vi "Parameter.vi"(5 "继承模式":string, 7 "模式":enum16{"select", "insert", "update", "delete"}(ring), 8 "nameData":T2(array[cluster]), 10 "parameterName":string, 11 "productsName":string) -> (0 "data":string[][](array[string]))   [LabVIEW 2013]
uses:
  <vilib>/Utility/VariantDataType/Type.ctl
  <vilib>/addons/database/_DB Variant To Data/Database Variant To Data.xnode
  <vilib>/Utility/VariantDataType/VariantType.lvlib
panel:
  out "SQL query":string
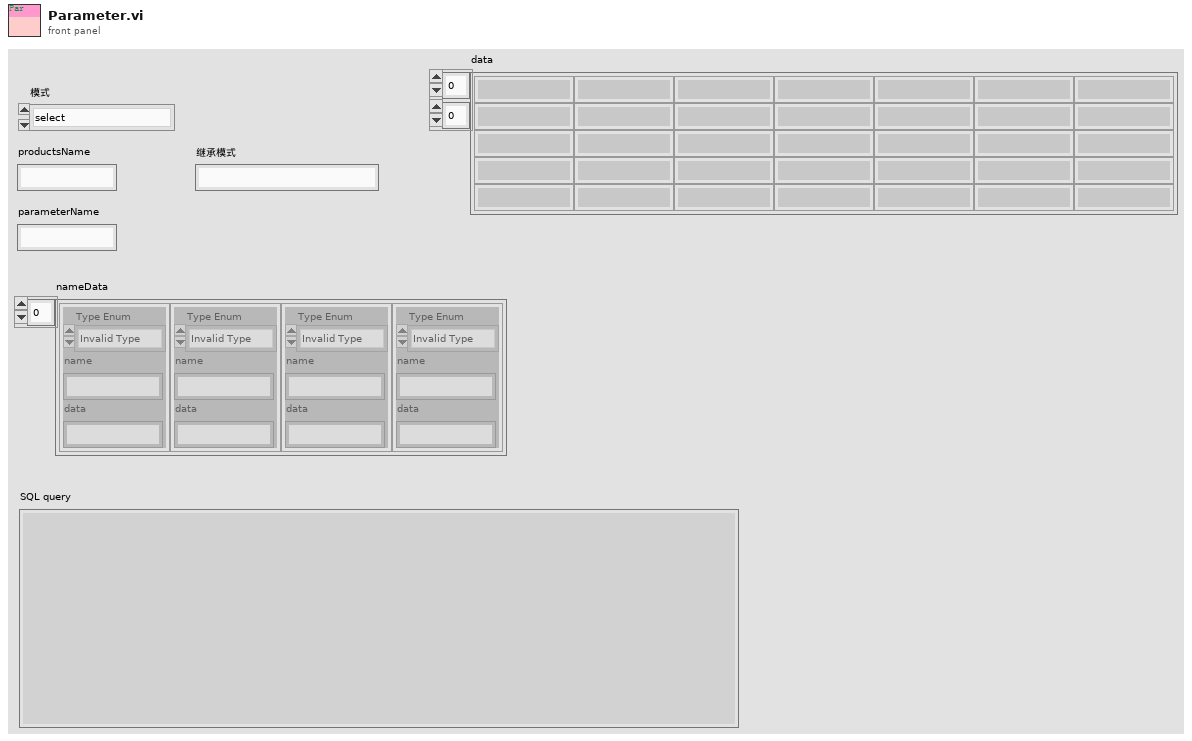
[diagram p1: front panel]
types:
  T1 = typedef "VariantType.lvlib/Type.ctl" = enum8{"Invalid Type", "Void", "I8", "I16", "I32", "I64", "U8", "U16", "U32", "U64", "Single Float", "Double Float", "Extended Float", "Single Complex", "Double Complex", "Extended Complex", "Enum U8", "Enum U16", "Enum U32", "Enum U64", "Single Float With Unit", "Double Float With Unit", "Extended Float With Unit", "Single Complex with Unit", "Double Complex with Unit", "Extended Complex with Unit", "Boolean", "String", "Path", "Picture", "Tag", "Array", "Cluster", "Variant", "LV Variant", "Waveform", "Timestamp", "Digital Waveform", "Digital Data", "ExpressData", "Refnum", "External Data", "VI", "Poly VI", "LabVIEW Class Instance", "Fixed Point"}
  T2 = cluster{"Type Enum":T1, "name":string, "data":string}[]
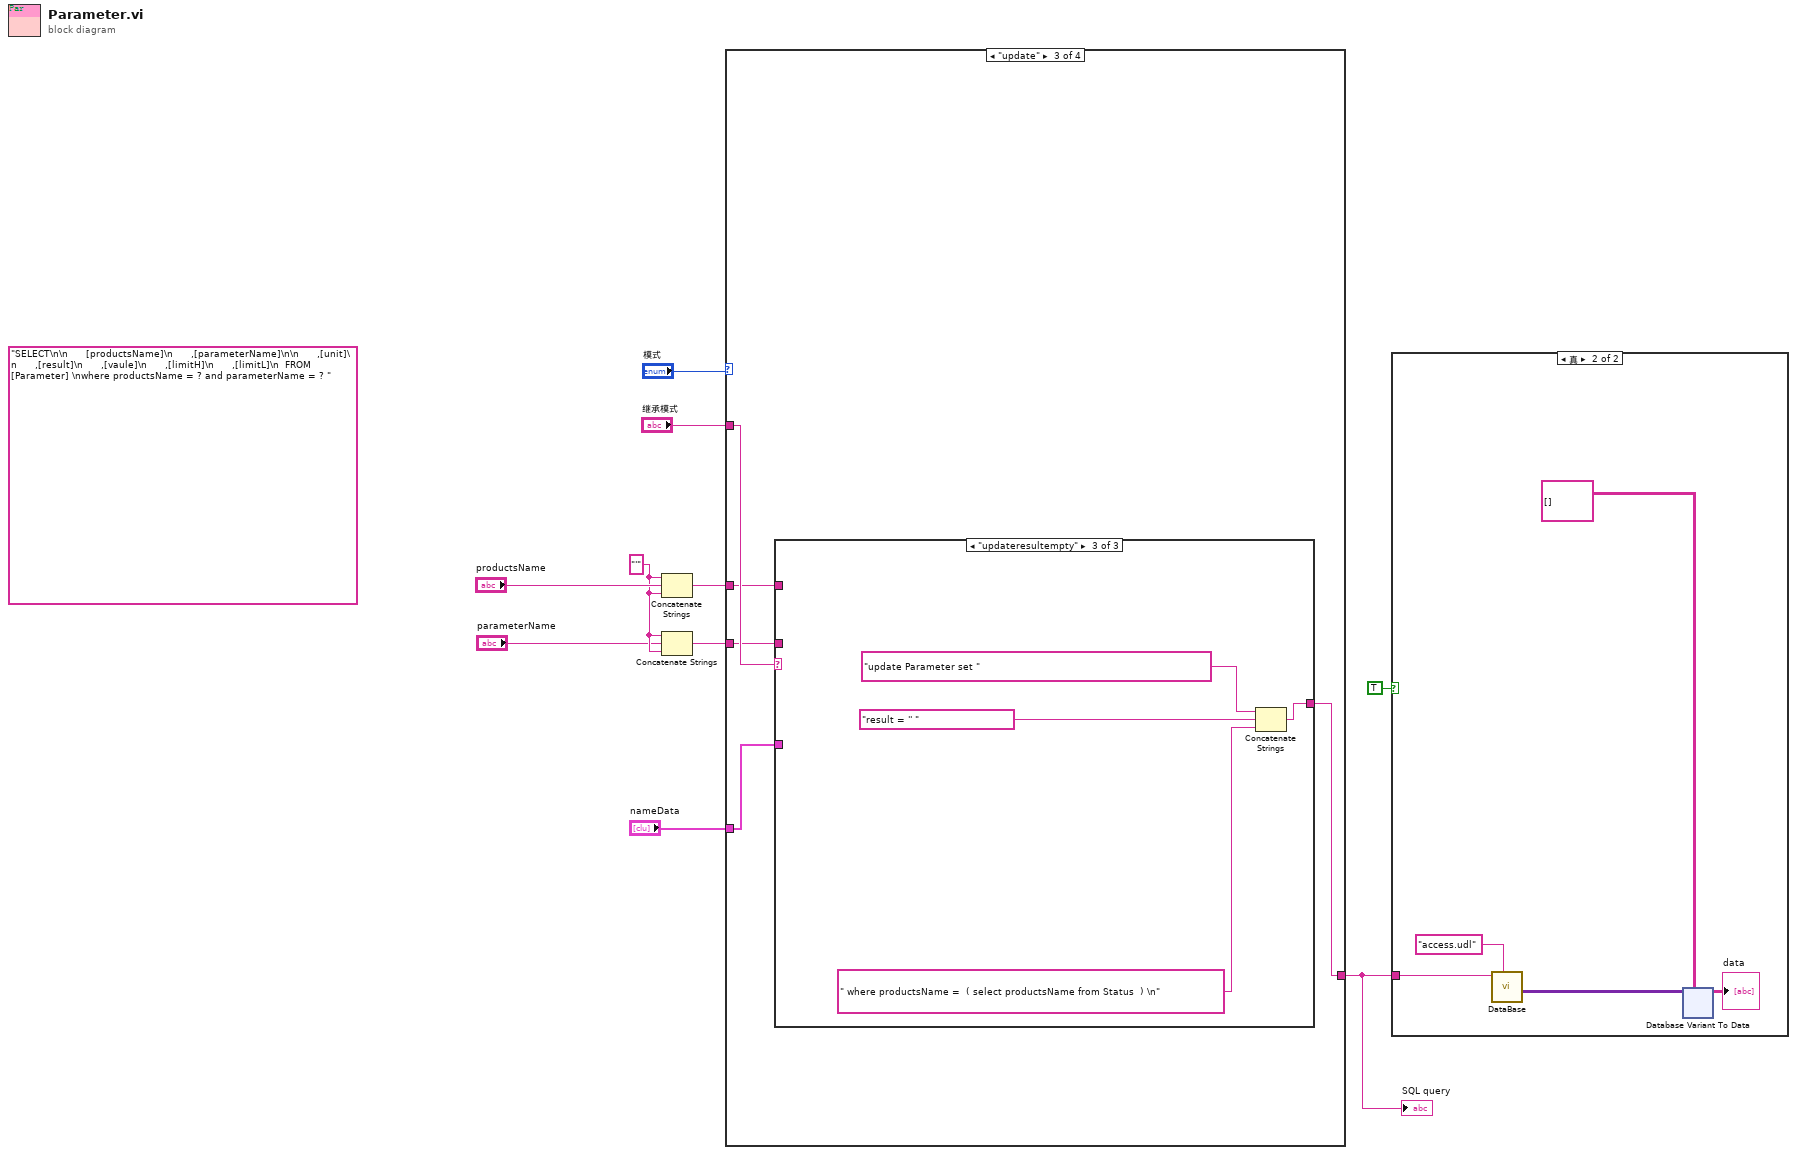
[diagram p0: block diagram]
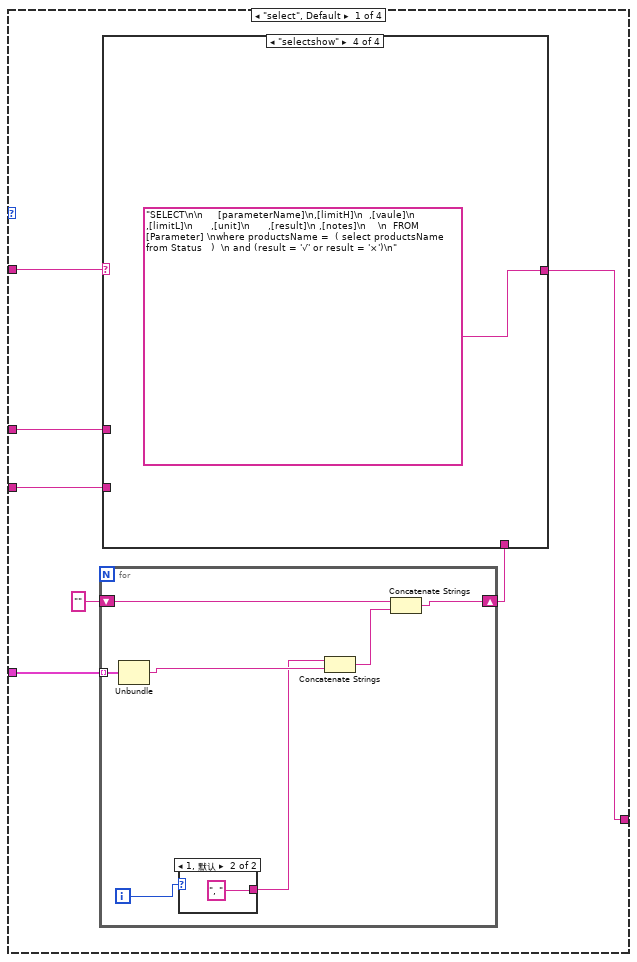
[diagram p3: hidden frame]
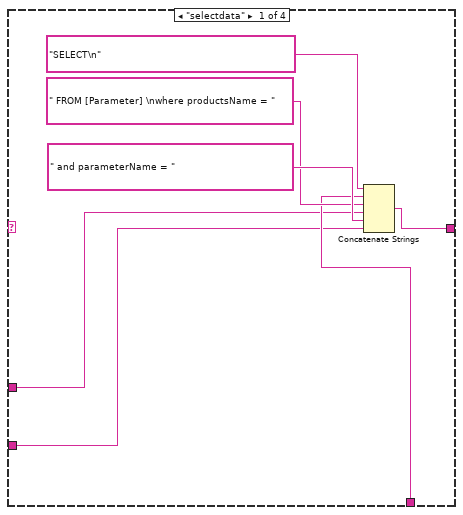
[diagram p4: hidden frame]
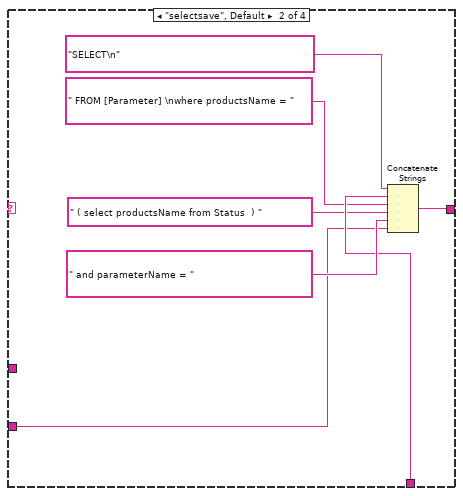
[diagram p5: hidden frame]
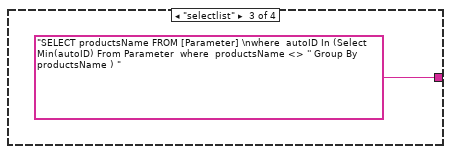
[diagram p6: hidden frame]
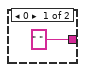
[diagram p7: hidden frame]
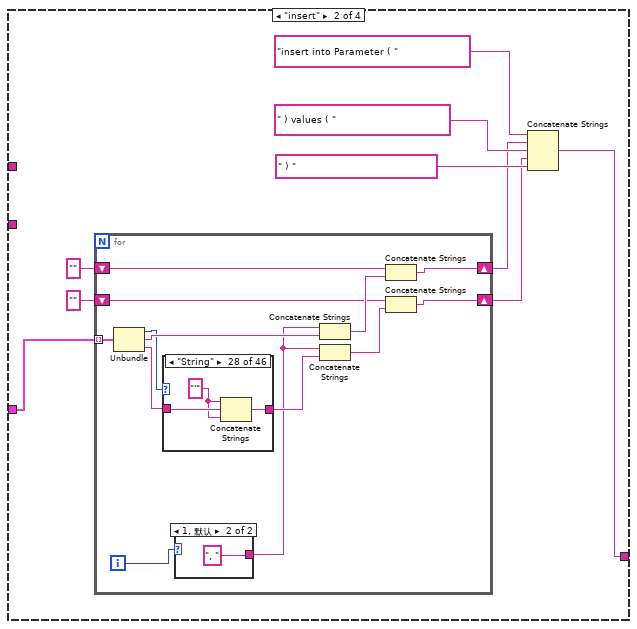
[diagram p8: hidden frame]
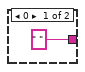
[diagram p9: hidden frame]
diagram:
  w4 = "'" ("字符串")
  (unwired) "SELECT\n\n      [productsName]\n      ,[parameterName]\n\n      ,[unit]\n      ,[result]\n      ,[vaule]\n      ,[limitH]\n      ,[limitL]\n  FROM [Parameter] \nwhere productsName = ? and parameterName = ? " ("SQL query")
  n1 = Concatenate Strings(w4, "productsName", w4) -> (w6:string)
  n2 = Concatenate Strings(w4, "parameterName", w4) -> (w2:string)
  n3 = case shown="\"update\"" "模式" {
    tunnel: [w11 w43 w77 w137] -> w9
    tunnel: "nameData" -> [w16 w49 w76 _]
    tunnel: w6 -> [w13 _ w73 w138]
    tunnel: w2 -> [w12 _ w74 _]
    tunnel: "继承模式" -> [w15 _ w75 _]
    frame "select", Default {
      n4 = for {
        tunnel: w16 -> [w40] mode=indexing
        shift-right: [w38] -> w14
        shift-left: "" ("SQL query") -> [w39]
        i -> [w35]
        n5 = Unbundle(w40) -> ("name"=w36:string)  [unwired: 2 out]
        n6 = case shown="1, 默认" w35 {
          tunnel: [" " ("字符串") ", " ("字符串")] -> w34
          frame 0 {
          }
          frame 1, Default {
          }
        }
        n7 = Concatenate Strings(w34, w36) -> (w37:string)
        n8 = Concatenate Strings(w39, w37) -> (w38:string)
      }
      n9 = case shown="\"selectshow\"" w15 {
        tunnel: [w18 w25 "SELECT productsName FROM [Parameter] \nwhere  autoID In (Select Min(autoID) From Parameter  where  productsName <> '' Group By productsName ) " ("SQL query") "SELECT\n\n     [parameterName]\n,[limitH]\n  ,[vaule]\n      ,[limitL]\n      ,[unit]\n      ,[result]\n ,[notes]\n    \n  FROM [Parameter] \nwhere productsName =  ( select productsName from Status   )  \n and (result = '√' or result = '×')\n" ("SQL query")] -> w11
        tunnel: w14 -> [w21 w29 _ _]
        tunnel: w13 -> [w20 _ _ _]
        tunnel: w12 -> [w19 w26 _ _]
        frame "selectdata" {
          n10 = Concatenate Strings("SELECT\n" ("SQL query"), w21, " FROM [Parameter] \nwhere productsName = " ("SQL query"), w20, " and parameterName = " ("SQL query"), w19) -> (w18:string)
        }
        frame "selectsave", Default {
          n11 = Concatenate Strings("SELECT\n" ("SQL query"), w29, " FROM [Parameter] \nwhere productsName = " ("SQL query"), " ( select productsName from Status  ) " ("SQL query"), " and parameterName = " ("SQL query"), w26) -> (w25:string)
        }
        frame "selectlist" {
        }
        frame "selectshow" {
        }
      }
    }
    frame "insert" {
      n12 = for {
        tunnel: w49 -> [w64] mode=indexing
        shift-right: [w62] -> w45
        shift-left: "" ("SQL query") -> [w63]
        shift-right: [w59] -> w44
        shift-left: "" ("SQL query") -> [w60]
        i -> [w53]
        n13 = Unbundle(w64) -> ("Type Enum"=w56:T1, "name"=w57:string, "data"=w55:string)
        n14 = case shown="\"String\"" w56 {
          tunnel: w55 -> [w67 _ _ _ _ _ _ _ _ _ w68 w69 _ _ _ _ _ _ _ _ _ _ _ _ _ _ _ w72 _ _ _ _ _ _ _ _ _ _ _ _ _ _ _ _ _ _]
          tunnel: [w67 _ _ _ _ _ _ _ _ _ w68 w69 _ _ _ _ _ _ _ _ _ _ _ _ _ _ _ w70 _ _ _ _ _ _ _ _ _ _ _ _ _ _ _ _ _ _] -> w54
          frame "Invalid Type", Default {
          }
          frame "Void" {
          }
          frame "I8" {
          }
          frame "I16" {
          }
          frame "I32" {
          }
          frame "I64" {
          }
          frame "U8" {
          }
          frame "U16" {
          }
          frame "U32" {
          }
          frame "U64" {
          }
          frame "Single Float" {
          }
          frame "Double Float" {
          }
          frame "Extended Float" {
          }
          frame "Single Complex" {
          }
          frame "Double Complex" {
          }
          frame "Extended Complex" {
          }
          frame "Enum U8" {
          }
          frame "Enum U16" {
          }
          frame "Enum U32" {
          }
          frame "Enum U64" {
          }
          frame "Single Float With Unit" {
          }
          frame "Double Float With Unit" {
          }
          frame "Extended Float With Unit" {
          }
          frame "Single Complex with Unit" {
          }
          frame "Double Complex with Unit" {
          }
          frame "Extended Complex with Unit" {
          }
          frame "Boolean" {
          }
          frame "String" {
            w71 = "'" ("字符串")
            n15 = Concatenate Strings(w71, w72, w71) -> (w70:string)
          }
          frame "Path" {
          }
          frame "Picture" {
          }
          frame "Tag" {
          }
          frame "Array" {
          }
          frame "Cluster" {
          }
          frame "Variant" {
          }
          frame "LV Variant" {
          }
          frame "Waveform" {
          }
          frame "Timestamp" {
          }
          frame "Digital Waveform" {
          }
          frame "Digital Data" {
          }
          frame "ExpressData" {
          }
          frame "Refnum" {
          }
          frame "External Data" {
          }
          frame "VI" {
          }
          frame "Poly VI" {
          }
          frame "LabVIEW Class Instance" {
          }
          frame "Fixed Point" {
          }
        }
        n16 = case shown="1, 默认" w53 {
          tunnel: [" " ("字符串") ", " ("字符串")] -> w52
          frame 0 {
          }
          frame 1, Default {
          }
        }
        n17 = Concatenate Strings(w52, w57) -> (w61:string)
        n18 = Concatenate Strings(w52, w54) -> (w58:string)
        n19 = Concatenate Strings(w63, w61) -> (w62:string)
        n20 = Concatenate Strings(w60, w58) -> (w59:string)
      }
      n21 = Concatenate Strings("insert into Parameter ( " ("SQL query"), w45, " ) values ( " ("SQL query"), w44, " ) " ("SQL query")) -> (w43:string)
    }
    frame "update" {
      n22 = case shown="\"updateresultempty\"" w75 {
        tunnel: [w82 w113 w136] -> w77
        tunnel: w76 -> [w81 w110 _]
        tunnel: w74 -> [w78 w107 _]
        tunnel: w73 -> [w80 _ _]
        frame "updatedata" {
          n23 = for {
            tunnel: w81 -> [w91] mode=indexing
            shift-right: [w96] -> w85
            shift-left: "" -> [w97]
            i -> [w88]
            n24 = Unbundle(w91) -> ("Type Enum"=w93:T1, "name"=w90:string, "data"=w92:string)
            n25 = case shown="\"String\"" w93 {
              tunnel: w92 -> [w100 _ _ _ _ _ _ _ _ _ w101 w102 _ _ _ _ _ _ _ _ _ _ _ _ _ _ _ w105 _ _ _ _ _ _ _ _ _ _ _ _ _ _ _ _ _ _]
              tunnel: [w100 _ _ _ _ _ _ _ _ _ w101 w102 _ _ _ _ _ _ _ _ _ _ _ _ _ _ _ w103 _ _ _ _ _ _ _ _ _ _ _ _ _ _ _ _ _ _] -> w89
              frame "Invalid Type", Default {
              }
              frame "Void" {
              }
              frame "I8" {
              }
              frame "I16" {
              }
              frame "I32" {
              }
              frame "I64" {
              }
              frame "U8" {
              }
              frame "U16" {
              }
              frame "U32" {
              }
              frame "U64" {
              }
              frame "Single Float" {
              }
              frame "Double Float" {
              }
              frame "Extended Float" {
              }
              frame "Single Complex" {
              }
              frame "Double Complex" {
              }
              frame "Extended Complex" {
              }
              frame "Enum U8" {
              }
              frame "Enum U16" {
              }
              frame "Enum U32" {
              }
              frame "Enum U64" {
              }
              frame "Single Float With Unit" {
              }
              frame "Double Float With Unit" {
              }
              frame "Extended Float With Unit" {
              }
              frame "Single Complex with Unit" {
              }
              frame "Double Complex with Unit" {
              }
              frame "Extended Complex with Unit" {
              }
              frame "Boolean" {
              }
              frame "String" {
                w104 = "'" ("字符串")
                n26 = Concatenate Strings(w104, w105, w104) -> (w103:string)
              }
              frame "Path" {
              }
              frame "Picture" {
              }
              frame "Tag" {
              }
              frame "Array" {
              }
              frame "Cluster" {
              }
              frame "Variant" {
              }
              frame "LV Variant" {
              }
              frame "Waveform" {
              }
              frame "Timestamp" {
              }
              frame "Digital Waveform" {
              }
              frame "Digital Data" {
              }
              frame "ExpressData" {
              }
              frame "Refnum" {
              }
              frame "External Data" {
              }
              frame "VI" {
              }
              frame "Poly VI" {
              }
              frame "LabVIEW Class Instance" {
              }
              frame "Fixed Point" {
              }
            }
            n27 = case shown="1, 默认" w88 {
              tunnel: [" " ("字符串") ", " ("字符串")] -> w87
              frame 0 {
              }
              frame 1, Default {
              }
            }
            n28 = Concatenate Strings(w87, w90, " = " ("SQL query"), w89) -> (w94:string)
            n29 = Concatenate Strings(w97, w94) -> (w96:string)
          }
          n30 = Concatenate Strings("update Parameter set " ("SQL query"), w85, "  where productsName = " ("SQL query"), w80, " and parameterName = " ("SQL query"), w78) -> (w82:string)
        }
        frame "updatesave", Default {
          n31 = for {
            N: 2 -> [_]
            tunnel: w110 -> [w118] mode=indexing
            shift-right: [w123] -> w109
            shift-left: "" -> [w124]
            i -> [w115]
            n32 = Unbundle(w118) -> ("Type Enum"=w120:T1, "name"=w117:string, "data"=w119:string)
            n33 = case shown="\"String\"" w120 {
              tunnel: w119 -> [w127 _ _ _ _ _ _ _ _ _ w128 w129 _ _ _ _ _ _ _ _ _ _ _ _ _ _ _ w132 _ _ _ _ _ _ _ _ _ _ _ _ _ _ _ _ _ _]
              tunnel: [w127 _ _ _ _ _ _ _ _ _ w128 w129 _ _ _ _ _ _ _ _ _ _ _ _ _ _ _ w130 _ _ _ _ _ _ _ _ _ _ _ _ _ _ _ _ _ _] -> w116
              frame "Invalid Type", Default {
              }
              frame "Void" {
              }
              frame "I8" {
              }
              frame "I16" {
              }
              frame "I32" {
              }
              frame "I64" {
              }
              frame "U8" {
              }
              frame "U16" {
              }
              frame "U32" {
              }
              frame "U64" {
              }
              frame "Single Float" {
              }
              frame "Double Float" {
              }
              frame "Extended Float" {
              }
              frame "Single Complex" {
              }
              frame "Double Complex" {
              }
              frame "Extended Complex" {
              }
              frame "Enum U8" {
              }
              frame "Enum U16" {
              }
              frame "Enum U32" {
              }
              frame "Enum U64" {
              }
              frame "Single Float With Unit" {
              }
              frame "Double Float With Unit" {
              }
              frame "Extended Float With Unit" {
              }
              frame "Single Complex with Unit" {
              }
              frame "Double Complex with Unit" {
              }
              frame "Extended Complex with Unit" {
              }
              frame "Boolean" {
              }
              frame "String" {
                w131 = "'" ("字符串")
                n34 = Concatenate Strings(w131, w132, w131) -> (w130:string)
              }
              frame "Path" {
              }
              frame "Picture" {
              }
              frame "Tag" {
              }
              frame "Array" {
              }
              frame "Cluster" {
              }
              frame "Variant" {
              }
              frame "LV Variant" {
              }
              frame "Waveform" {
              }
              frame "Timestamp" {
              }
              frame "Digital Waveform" {
              }
              frame "Digital Data" {
              }
              frame "ExpressData" {
              }
              frame "Refnum" {
              }
              frame "External Data" {
              }
              frame "VI" {
              }
              frame "Poly VI" {
              }
              frame "LabVIEW Class Instance" {
              }
              frame "Fixed Point" {
              }
            }
            n35 = case shown="1, 默认" w115 {
              tunnel: [" " ("字符串") ", " ("字符串")] -> w114
              frame 0 {
              }
              frame 1, Default {
              }
            }
            n36 = Concatenate Strings(w114, w117, " = " ("SQL query"), w116) -> (w121:string)
            n37 = Concatenate Strings(w124, w121) -> (w123:string)
          }
          n38 = Concatenate Strings("update Parameter set " ("SQL query"), w109, " where productsName =  ( select productsName from Status  ) \n and parameterName = " ("SQL query"), w107) -> (w113:string)
        }
        frame "updateresultempty" {
          n39 = Concatenate Strings("update Parameter set " ("SQL query"), "result = '' ", " where productsName =  ( select productsName from Status  ) \n" ("SQL query")) -> (w136:string)
        }
      }
    }
    frame "delete" {
      n40 = Concatenate Strings("delete  from Parameter where  productsName =  \n" ("SQL query"), w138) -> (w137:string)
    }
  }
  "SQL query" <- w9
  n41 = case shown="真" TRUE {
    tunnel: w9 -> [_ w142]
    frame False {
    }
    frame True {
      n42 = call "DataBase.vi"("udl名称"="access.udl", "SQL query"=w142) -> ("recordset data"=w144:variant[][])  [unwired: 9 in]
      n43 = xnode ("Database Variant To Data")("database variant"=w144, "type"=string[][] [] ("添加的数组")) -> ("data"=→"data":string[][])  [unwired: 1 in, 1 out]
    }
  }
